vi "Read Image Size.vi"(8 "error in (no error)":errorcluster, 11 "Image Distorter in":refnum<class "Image Distorter.lvclass">) -> (0 "error out":errorcluster, 2 "Image Size":T1, 3 "Image Distorter":refnum<class "Image Distorter.lvclass">)   [LabVIEW 2020, in "ar.lvlib" / "Image Distorter.lvclass"]
doc: "Get the Image Size that the Image Distorter has been configured for."
uses:
  Image Distorter.lvclass
  common/Image Size (Integer).ctl
  Image Distorter.lvclass/Image Distorter.ctl
  common/common.lvlib
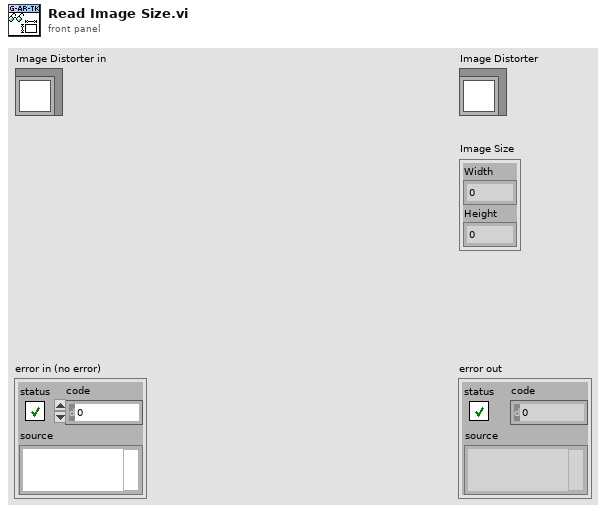
[diagram p1: front panel]
types:
  T1 = typedef "common.lvlib/Image Size (Integer).ctl" = cluster{"Width":u16, "Height":u16}
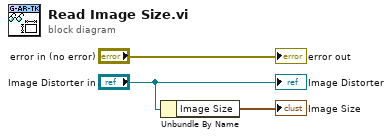
[diagram p0: block diagram]
diagram:
  n1 = Unbundle By Name("Image Distorter in") -> ("Image Size"=→"Image Size":T1)
  "error out" <- "error in (no error)"
  "Image Distorter" <- "Image Distorter in"
